vi "Hysteresis_Math.vi"(8 "Discesa":dbl[][](array[numeric]), 10 "Salita":dbl[][](array[numeric])) -> (0 "Max Delta":dbl, 1 "Maximum uncertainty Descending Phase":dbl, 2 "Maximum uncertainty Ascending Phase":dbl, 3 "abs_DELTA point-by-point":dbl[](array[numeric]), 4 "uncertainty ascending phase (point-by-point)":dbl[](array[numeric]), 5 "aithmetical mean descending phase":dbl[](array[numeric]), 6 "uncertainty descending phase (point-by-point)":dbl[](array[numeric]), 7 "arithmetical mean acending phase":dbl[](array[numeric]))   [LabVIEW 2021, in "CALIBRATION.lvlib"]
uses:
  CALIBRATION.lvlib
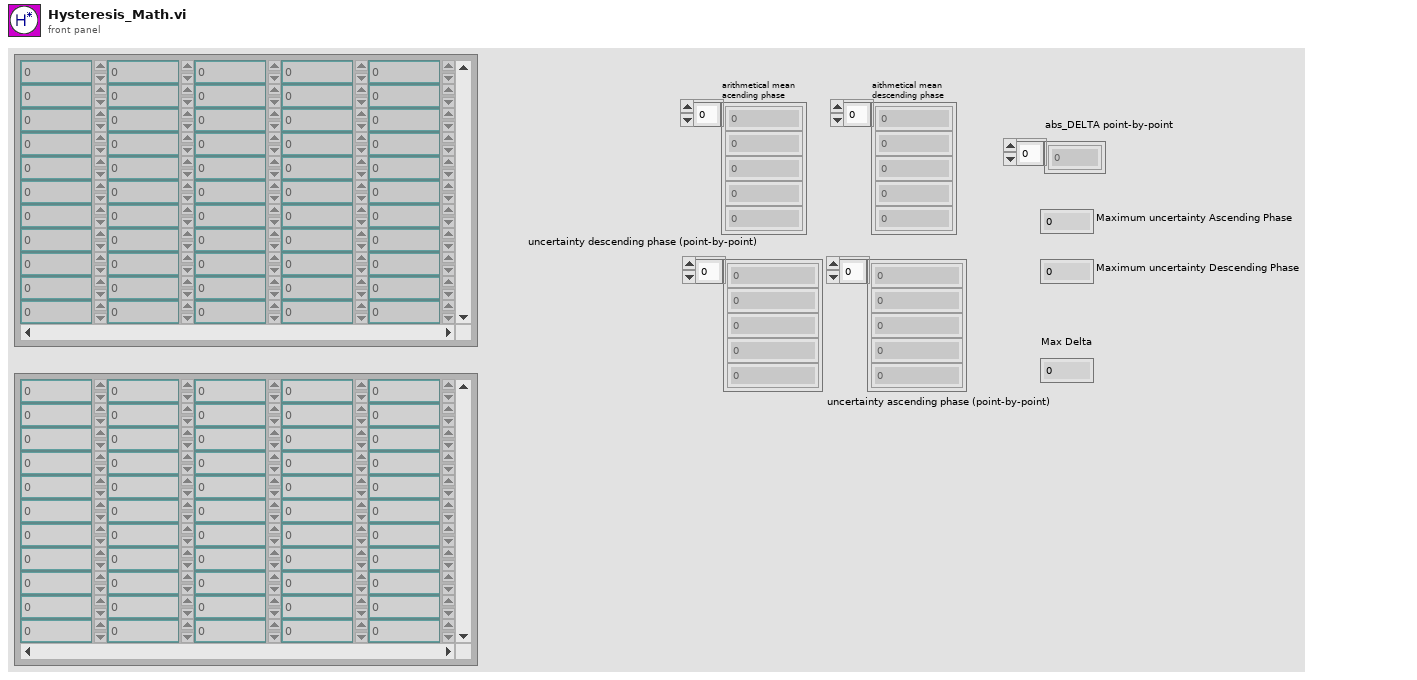
[diagram p1: front panel]
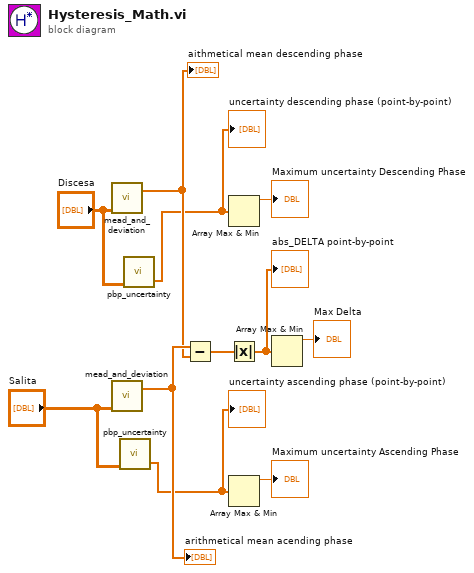
[diagram p0: block diagram]
diagram:
  n1 = call "mead_and_deviation.vi"("insieme"="Discesa") -> ("Media"=w10:dbl[])  [unwired: 3 in, 1 out]
  "aithmetical mean descending phase" <- w10
  n2 = call "mead_and_deviation.vi"("insieme"="Salita") -> ("Media"=w11:dbl[])  [unwired: 3 in, 1 out]
  "arithmetical mean acending phase" <- w11
  n3 = call "pbp_uncertainty.vi"("insieme"="Salita") -> ("Incertezza"=w2:dbl[])  [unwired: 4 in]
  "uncertainty ascending phase (point-by-point)" <- w2
  n4 = call "pbp_uncertainty.vi"("insieme"="Discesa") -> ("Incertezza"=w1:dbl[])  [unwired: 4 in]
  "uncertainty descending phase (point-by-point)" <- w1
  n5 = Subtract(x=w11, y=w10) -> (x-y=w9:dbl[])
  n6 = Array Max & Min(array=w1) -> (max value=→"Maximum uncertainty Descending Phase":dbl)  [unwired: 3 out]
  n7 = Absolute Value(x=w9) -> (abs(x)=w8:dbl[])
  "abs_DELTA point-by-point" <- w8
  n8 = Array Max & Min(array=w2) -> (max value=→"Maximum uncertainty Ascending Phase":dbl)  [unwired: 3 out]
  n9 = Array Max & Min(array=w8) -> (max value=→"Max Delta":dbl)  [unwired: 3 out]
